vi "Get ParameterName+.vi"(8 "Error In":errorcluster, 11 "reference in":refnum<class "OD Entry.lvclass">) -> (0 "Error Out":errorcluster, 1 "Defined?":bool, 2 "ParameterName":string, 3 "reference out":refnum<class "OD Entry.lvclass">)   [LabVIEW 2019, in "Electronic Datasheet.lvlib" / "OD Entry.lvclass"]
uses:
  OD Entry.lvclass
  Object Type/Object Type Base.lvclass
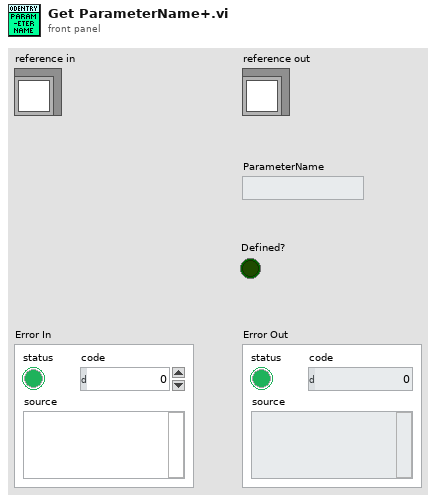
[diagram p1: front panel]
types:
  T1 = typedef "Electronic Datasheet.lvlib/OD Entry.lvclass/ObjectAttributes.ctl" = cluster{"Index":u16, "ObjectType":refnum<class "Object Type Base.lvclass">, "Denotation":string, "Count":u8, "ObjExtend":u8, "Label":string, "Description":string, "PDO Mapping Type":T2, "Sub-Entries":map{u8, refnum<class "OD Sub-Entry.lvclass">}}
  T2 = typedef "Electronic Datasheet.lvlib/PDO Mapping Type.ctl" = enum16{"no", "optional", "RPDO", "TPDO", "UNKNOWN"}
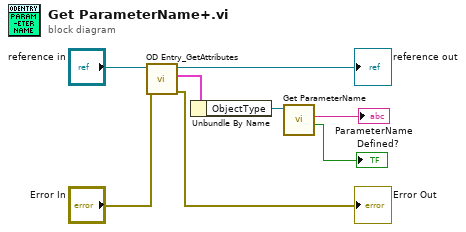
[diagram p0: block diagram]
diagram:
  n1 = call "OD Entry_GetAttributes.vi"("Error In"="Error In", "reference in"="reference in") -> ("Error Out"=→"Error Out":errorcluster, "Data"=w5:T1, "reference out"=→"reference out":refnum<class "OD Entry.lvclass">)  [unwired: 6 in, 1 out]
  n2 = Unbundle By Name(w5) -> ("ObjectType"=w4:refnum<class "Object Type Base.lvclass">)
  n3 = call "Get ParameterName.vi"("Object Type in"=w4) -> ("Defined?"=→"Defined?":bool, "ParameterName"=→"ParameterName":string)  [unwired: 8 in, 1 out]
